vi "Update Waveform.vi"(8 "error in (no error)":errorcluster, 10 "Waveform":refnum<class "Waveform.lvclass">, 11 "Channel in":refnum<class "Channel.lvclass">) -> (0 "error out":errorcluster, 3 "Channel out":refnum<class "Channel.lvclass">)   [LabVIEW 2015, in "Channel.lvclass"]
uses:
  Channel.lvclass
  Waveforms/Waveform/Waveform.lvclass
  Channel.lvclass/Channel.ctl
  Modulations/AM/AM.lvclass
  Filter/Filter.lvclass
  Koop/KObject Class/KObject.lvclass
panel:
  out "Waveshape changed":bool
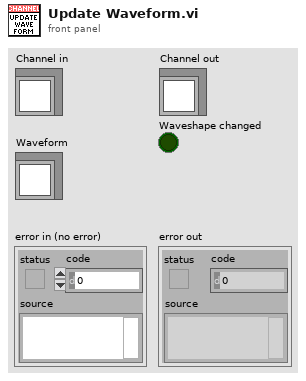
[diagram p1: front panel]
types:
  T1 = typedef "Waveform.lvclass/Attributes.ctl" = cluster{"Spectrum":bool, "Gate":bool, "Mod":bool, "Filter":bool}
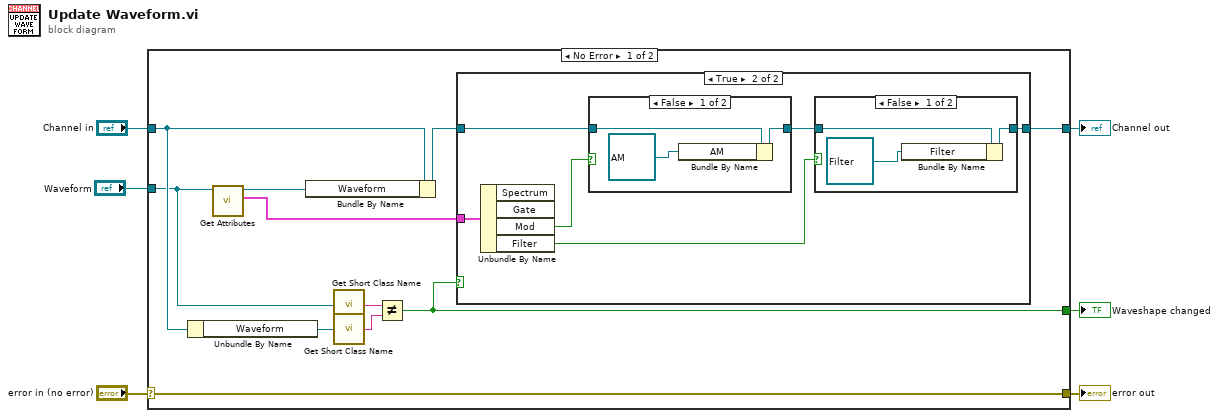
[diagram p0: block diagram]
diagram:
  n1 = case shown="No Error" "error in (no error)" {
    selector: "error in (no error)" -> [w17 w34]
    tunnel: [w17 w34] -> w5
    tunnel: [w10 w33] -> w3
    tunnel: "Channel in" -> [w16 w33]
    tunnel: "Waveform" -> [w9 _]
    tunnel: [w12 _] -> w1
    frame No Error {
      n2 = Unbundle By Name(w16) -> ("Waveform"=w15:refnum<class "Waveform.lvclass">)
      n3 = call-dynamic "Get Attributes.vi"("Waveform in"=w9) -> ("Attributes"=w7:T1, "Waveform out"=w8:refnum<class "Waveform.lvclass">)  [unwired: 8 in, 1 out]
      n4 = Bundle By Name(cluster=w16, "Waveform"=w8) -> (w11:refnum<class "Channel.lvclass">)
      n5 = call "Get Short Class Name.vi"("KObject in"=w9) -> ("Class"=w14:string)  [unwired: 4 in]
      n6 = call "Get Short Class Name.vi"("KObject in"=w15) -> ("Class"=w13:string)  [unwired: 4 in]
      n7 = Not Equal?(x=w14, y=w13) -> (x != y?=w12:bool)
      n8 = case shown="True" w12 {
        tunnel: w11 -> [w18 w22]
        tunnel: [w18 w20] -> w10
        tunnel: w7 -> [_ w24]
        frame False {
        }
        frame True {
          n9 = Unbundle By Name(w24) -> ("Mod"=w23:bool, "Filter"=w19:bool)  [unwired: 2 out]
          n10 = case shown="False" w23 {
            tunnel: w22 -> [w31 w32]
            tunnel: [w30 w32] -> w21
            frame False {
              n11 = Bundle By Name(cluster=w31, "AM"=refnum<class "AM.lvclass"> refnum ("Serialized.AM")) -> (w30:refnum<class "Channel.lvclass">)
            }
            frame True {
            }
          }
          n12 = case shown="False" w19 {
            tunnel: w21 -> [w27 w28]
            tunnel: [w26 w28] -> w20
            frame False {
              n13 = Bundle By Name(cluster=w27, "Filter"=refnum<class "Filter.lvclass"> refnum ("Serialized.Filter")) -> (w26:refnum<class "Channel.lvclass">)
            }
            frame True {
            }
          }
        }
      }
    }
    frame Error {
    }
  }
  "error out" <- w5
  "Channel out" <- w3
  "Waveshape changed" <- w1
